vi "Query Builder.vi"(8 "Date-Time Column Name":string="Date-Time", 9 "2nd Search Column Name":string=" Lot_ID ", 10 "1st Search Column Name":string=" CryoProber_MCT_Std_Sample_Summary.Sample_Name ", 11 "Query Build Cluster":T1={"Sample Check box"=TRUE, "Sample Comparison Type"="Is exactly", "Sample Name"="", "Logical Sample-Lot "="OR", "LotID Checkbox"=TRUE, "Lot Comparison Type"="Is exactly", "LotID Name"="", "Logical Lot-Date"="OR", "Date Checkbox"=TRUE, "Start Date"=timestamp(3375812149.928578 s since 1904-01-01), "End Date"=timestamp(3375812149.928578 s since 1904-01-01)} {"Start Date" format="%<%X\n%x>T"; "End Date" format="%<%X\n%x>T"}) -> (3 "Where Statement":string=" WHERE (  CryoProber_MCT_Std_Sample_Summary.Sample_Name  = '' OR  Lot_ID  = '' OR [Date-Time] BETWEEN CONVERT (Datetime, '12/21/2010 15:35:49') AND CONVERT (Datetime, '12/21/2010 15:35:49') ) ")   [LabVIEW 2010]
panel:
  # "Get all results where the VARNAME"
  # "where the VAR2"
  # "between these dates"
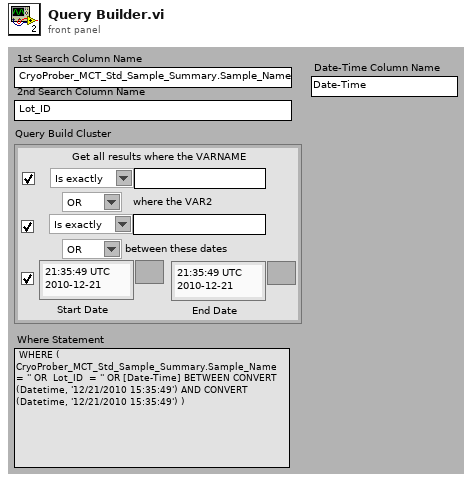
[diagram p1: front panel]
types:
  T1 = cluster{"Sample Check box":bool, "Sample Comparison Type":string, "Sample Name":string, "Logical Sample-Lot ":string, "LotID Checkbox":bool, "Lot Comparison Type":string, "LotID Name":string, "Logical Lot-Date":string, "Date Checkbox":bool, "Start Date":timestamp, "End Date":timestamp}
  T2 = enum16{"MS SQL Format", "Access Format", "Using CONVERT func", "Using # # "}
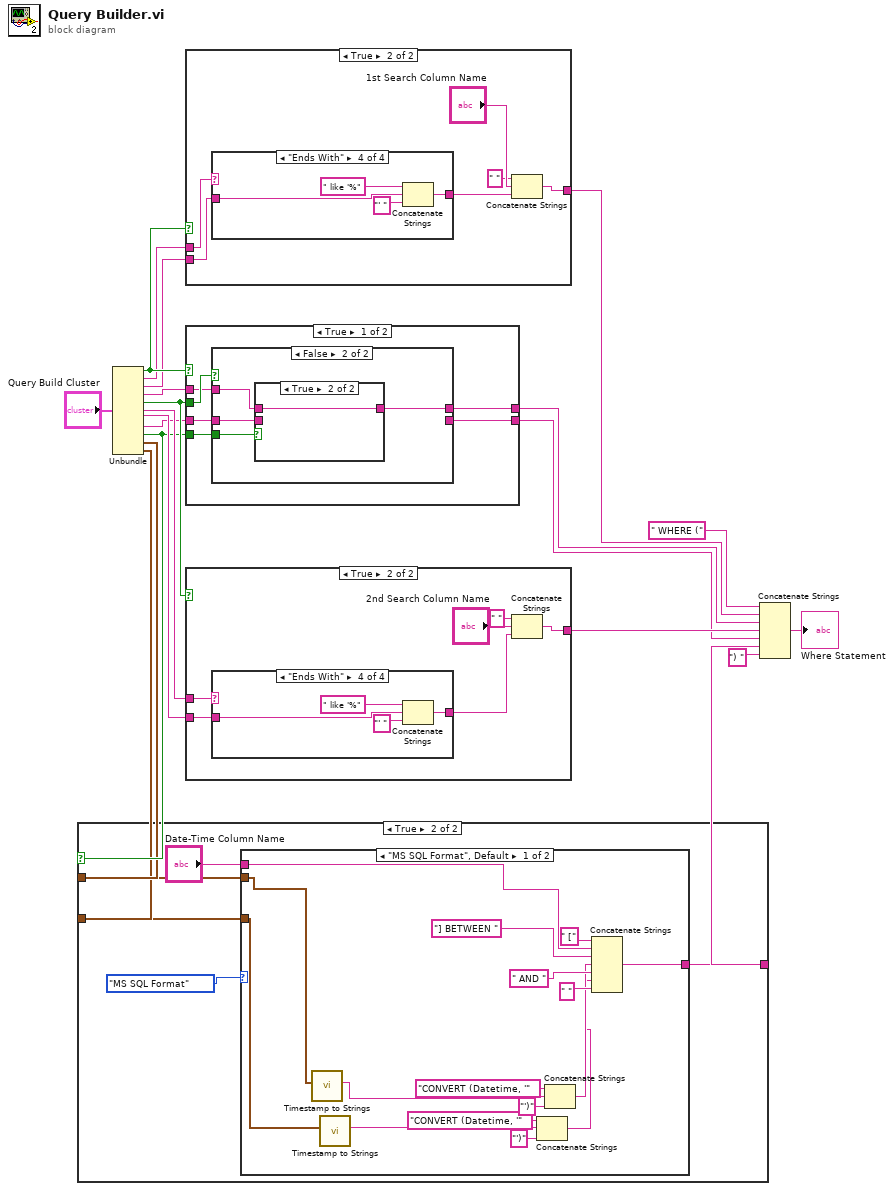
[diagram p0: block diagram]
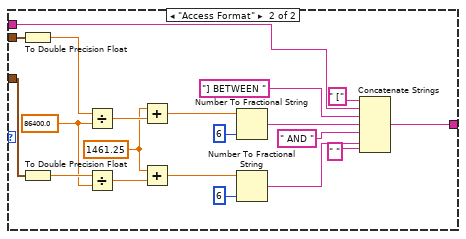
[diagram p3: hidden frame]
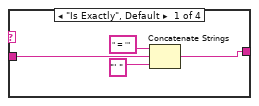
[diagram p5: hidden frame]
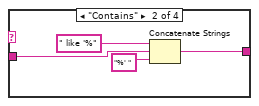
[diagram p6: hidden frame]
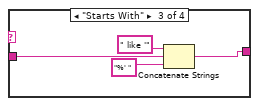
[diagram p7: hidden frame]
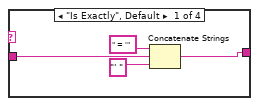
[diagram p9: hidden frame]
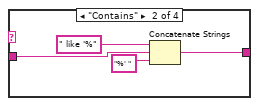
[diagram p10: hidden frame]
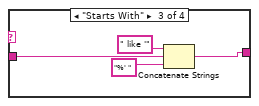
[diagram p11: hidden frame]
diagram:
  n1 = Unbundle("Query Build Cluster") -> ("Sample Check box"=w13:bool, "Sample Comparison Type"=w12:string, "Sample Name"=w11:string, "Logical Sample-Lot"=w10:string, "LotID Checkbox"=w9:bool, "Lot Comparison Type"=w8:string, "LotID Name"=w7:string, "Logical Lot-Date"=w6:string, "Date Checkbox"=w5:bool, "Start Date"=w4:timestamp, "End Date"=w3:timestamp)
  n2 = case shown="True" w5 {
    tunnel: [_ w25] -> w15
    tunnel: w4 -> [_ w23]
    tunnel: w3 -> [_ w24]
    frame False {
    }
    frame True {
      n3 = case shown="\"MS SQL Format\", Default" T2."MS SQL Format" {
        tunnel: [w38 w58] -> w25
        tunnel: w24 -> [w27 w56]
        tunnel: w23 -> [w31 w54]
        tunnel: "Date-Time Column Name" -> [w36 w42]
        frame "MS SQL Format", Default {
          n4 = call "Timestamp to Strings.vi"("Input Time"=w31) -> ("DB Date-Time"=w32:string)  [unwired: 3 in, 3 out]
          n5 = call "Timestamp to Strings.vi"("Input Time"=w27) -> ("DB Date-Time"=w26:string)  [unwired: 3 in, 3 out]
          n6 = Concatenate Strings("CONVERT (Datetime, '" ("string"), w26, "')" ("string")) -> (w28:string)
          n7 = Concatenate Strings("CONVERT (Datetime, '" ("string"), w32, "')" ("string")) -> (w33:string)
          n8 = Concatenate Strings(" [" ("string"), w36, "] BETWEEN " ("string"), w33, " AND " ("string"), w28, " " ("string")) -> (w38:string)
        }
        frame "Access Format" {
          w44 = 1461.25 ("x")
          w43 = 86400.0 ("y")
          n9 = To Double Precision Float(number=w54) -> (double precision float=w52:dbl)
          n10 = To Double Precision Float(number=w56) -> (double precision float=w51:dbl)
          n11 = Divide(x=w52, y=w43) -> (x/y=w55:dbl)
          n12 = Divide(x=w51, y=w43) -> (x/y=w53:dbl)
          n13 = Add(x=w44, y=w55) -> (x+y=w48:dbl)
          n14 = Add(x=w44, y=w53) -> (x+y=w47:dbl)
          n15 = Number To Fractional String(number=w48, precision (6)=i16 6) -> (F-format string=w46:string)  [unwired: 2 in]
          n16 = Number To Fractional String(number=w47, precision (6)=i16 6) -> (F-format string=w45:string)  [unwired: 2 in]
          n17 = Concatenate Strings(" [" ("string"), w42, "] BETWEEN " ("string"), w46, " AND " ("string"), w45, " " ("string")) -> (w58:string)
        }
      }
    }
  }
  n18 = case shown="True" w13 {
    tunnel: [_ w65] -> w19
    tunnel: w11 -> [_ w64]
    tunnel: w12 -> [_ w63]
    frame False {
    }
    frame True {
      n19 = case shown="\"Ends With\"" w63 {
        tunnel: [w69 w73 w77 w81] -> w66
        tunnel: w64 -> [w68 w72 w76 w80]
        frame "Is Exactly", Default {
          n20 = Concatenate Strings(" = '" ("string"), w68, "' " ("string")) -> (w69:string)
        }
        frame "Contains" {
          n21 = Concatenate Strings(" like '%" ("string"), w72, "%' " ("string")) -> (w73:string)
        }
        frame "Starts With" {
          n22 = Concatenate Strings(" like '" ("string"), w76, "%' " ("string")) -> (w77:string)
        }
        frame "Ends With" {
          n23 = Concatenate Strings(" like '%" ("string"), w80, "' " ("string")) -> (w81:string)
        }
      }
      n24 = Concatenate Strings(" " ("string"), "1st Search Column Name", w66) -> (w65:string)
    }
  }
  n25 = case shown="True" w13 {
    tunnel: w9 -> [w89 w104]
    tunnel: w5 -> [w88 w103]
    tunnel: w10 -> [w87 w102]
    tunnel: [w86 _] -> w18
    tunnel: w6 -> [w85 w101]
    tunnel: [w84 w100] -> w16
    frame True {
      n26 = case shown="False" w89 {
        tunnel: w88 -> [w93 w98]
        tunnel: w87 -> [w92 w96]
        tunnel: [w92 w95] -> w86
        tunnel: w85 -> [w91 w97]
        tunnel: [w90 _] -> w84
        frame True {
          n27 = case shown="True" w93 {
            tunnel: w91 -> [_ w94]
            tunnel: [_ w94] -> w90
            frame False {
            }
            frame True {
            }
          }
        }
        frame False {
          n28 = case shown="True" w98 {
            tunnel: w97 -> [_ _]
            tunnel: w96 -> [_ w99]
            tunnel: [_ w99] -> w95
            frame False {
            }
            frame True {
            }
          }
        }
      }
    }
    frame False {
      n29 = case shown="False" w104 {
        tunnel: w103 -> [w107 _]
        tunnel: w102 -> [_ _]
        tunnel: w101 -> [w106 _]
        tunnel: [w105 _] -> w100
        frame True {
          n30 = case shown="False" w107 {
            tunnel: w106 -> [_ w108]
            tunnel: [_ w108] -> w105
            frame False {
            }
            frame True {
            }
          }
        }
        frame False {
        }
      }
    }
  }
  n31 = case shown="True" w9 {
    tunnel: w8 -> [_ w114]
    tunnel: w7 -> [_ w113]
    tunnel: [_ w110] -> w17
    frame False {
    }
    frame True {
      n32 = case shown="\"Ends With\"" w114 {
        tunnel: [w116 w120 w124 w128] -> w111
        tunnel: w113 -> [w115 w119 w123 w127]
        frame "Is Exactly", Default {
          n33 = Concatenate Strings(" = '" ("string"), w115, "' " ("string")) -> (w116:string)
        }
        frame "Contains" {
          n34 = Concatenate Strings(" like '%" ("string"), w119, "%' " ("string")) -> (w120:string)
        }
        frame "Starts With" {
          n35 = Concatenate Strings(" like '" ("string"), w123, "%' " ("string")) -> (w124:string)
        }
        frame "Ends With" {
          n36 = Concatenate Strings(" like '%" ("string"), w127, "' " ("string")) -> (w128:string)
        }
      }
      n37 = Concatenate Strings(" " ("string"), "2nd Search Column Name", w111) -> (w110:string)
    }
  }
  n38 = Concatenate Strings(" WHERE (" ("string"), w19, w18, w17, w16, w15, ") " ("string")) -> (→"Where Statement":string)
